vi "PV DATA TYPE.vi"(4 "String in":string, 5 "Data Typ String in":string) -> (1 "Substring":string, 2 "PV Protocol Data out":string)   [LabVIEW 2015, in "Pfeiffer Vacuum.lvlib"]
uses:
  Pfeiffer Vacuum.lvlib
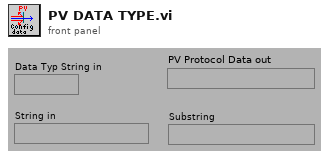
[diagram p1: front panel]
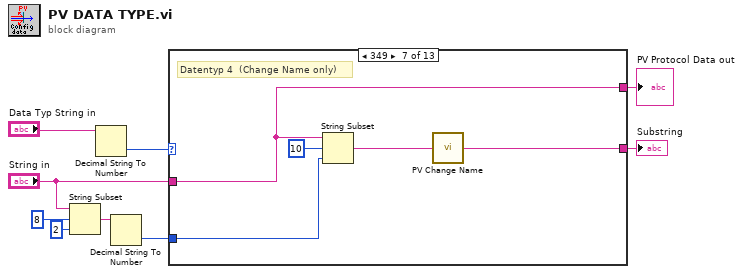
[diagram p0: block diagram]
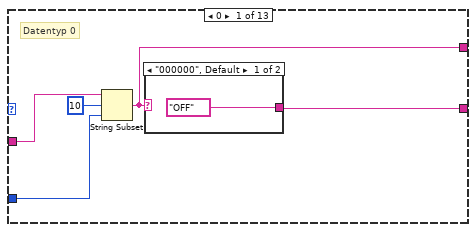
[diagram p2: hidden frame]
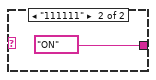
[diagram p3: hidden frame]
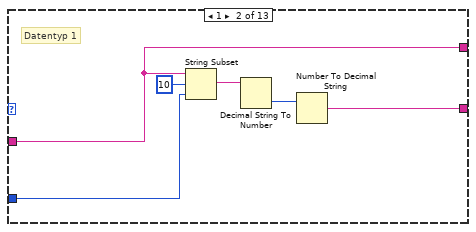
[diagram p4: hidden frame]
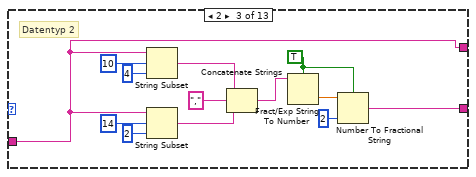
[diagram p5: hidden frame]
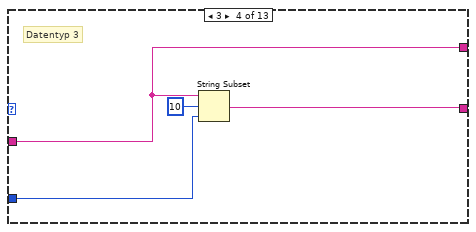
[diagram p6: hidden frame]
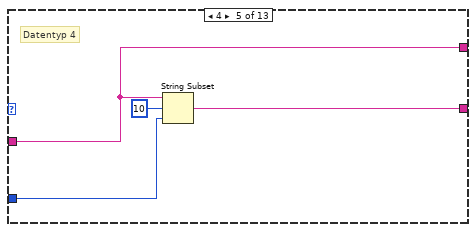
[diagram p7: hidden frame]
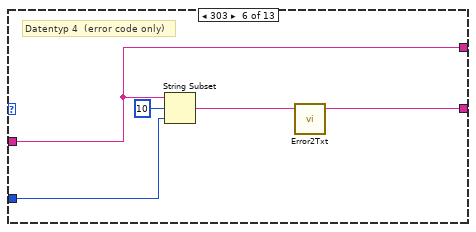
[diagram p8: hidden frame]
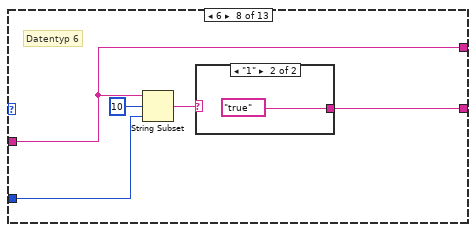
[diagram p9: hidden frame]
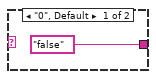
[diagram p10: hidden frame]
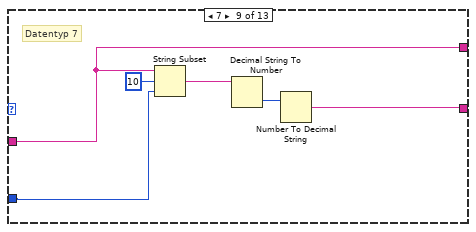
[diagram p11: hidden frame]
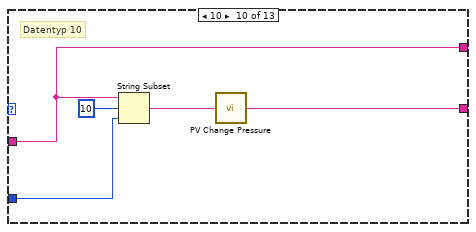
[diagram p12: hidden frame]
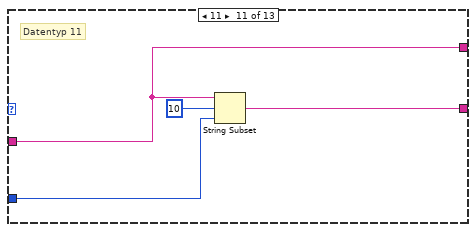
[diagram p13: hidden frame]
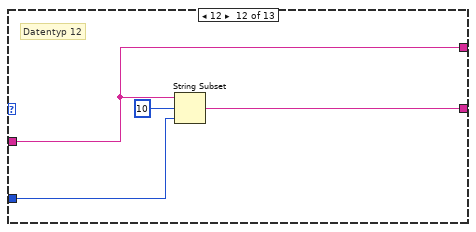
[diagram p14: hidden frame]
diagram:
  n1 = String Subset(string="String in", offset (0)=8 ("Offset (0)"), length (rest)=2 ("Länge (Rest)")) -> (substring=w4:string)
  n2 = Decimal String To Number(string="Data Typ String in") -> (number=w8:i32)  [unwired: 2 in, 1 out]
  n3 = Decimal String To Number(string=w4) -> (number=w2:i32)  [unwired: 2 in, 1 out]
  n4 = case shown="349" w8 {
    tunnel: "String in" -> [w12 w17 w23 w36 w40 w44 w49 w54 w61 w67 w72 w76 w80]
    tunnel: [w14 w21 w33 w38 w42 w46 w51 w56 w63 w69 w74 w77 w80] -> w9
    tunnel: w2 -> [w11 w18 _ w37 w41 w45 w50 w55 w62 w68 w73 w79 _]
    tunnel: [w10 w17 w23 w36 w40 w44 w49 w54 w61 w67 w72 w76 w80] -> w1
    frame 0 {
      # "Datentyp 0"
      n5 = String Subset(string=w12, offset (0)=10 ("Offset (0)"), length (rest)=w11) -> (substring=w10:string)
      n6 = case shown="\"000000\", Default" w10 {
        tunnel: ["OFF" "ON"] -> w14
        frame "000000", Default {
        }
        frame "111111" {
        }
      }
    }
    frame 1 {
      # "Datentyp 1"
      n7 = String Subset(string=w17, offset (0)=10 ("Offset (0)"), length (rest)=w18) -> (substring=w20:string)
      n8 = Decimal String To Number(string=w20) -> (number=w19:i32)  [unwired: 2 in, 1 out]
      n9 = Number To Decimal String(number=w19) -> (decimal integer string=w21:string)  [unwired: 1 in]
    }
    frame 2 {
      w24 = TRUE ("verwende System-Dezimalpunkt (T)")
      # "Datentyp 2"
      n10 = String Subset(string=w23, offset (0)=10 ("Offset (0)"), length (rest)=4 ("Länge")) -> (substring=w29:string)
      n11 = String Subset(string=w23, offset (0)=14 ("Offset (0)"), length (rest)=2 ("Länge")) -> (substring=w28:string)
      n12 = Concatenate Strings(w29, ",", w28) -> (w26:string)
      n13 = Fract/Exp String To Number(use system decimal point (T)=w24, string=w26) -> (number=w25:dbl)  [unwired: 2 in, 1 out]
      n14 = Number To Fractional String(use system decimal point (T)=w24, number=w25, precision (6)=i16 2 ("Genauigkeit (6)")) -> (F-format string=w33:string)  [unwired: 1 in]
    }
    frame 3 {
      # "Datentyp 3"
      n15 = String Subset(string=w36, offset (0)=10 ("Offset (0)"), length (rest)=w37) -> (substring=w38:string)
    }
    frame 4 {
      # "Datentyp 4"
      n16 = String Subset(string=w40, offset (0)=10 ("Offset (0)"), length (rest)=w41) -> (substring=w42:string)
    }
    frame 303 {
      # "Datentyp 4  (error code only)"
      n17 = String Subset(string=w44, offset (0)=10 ("Offset (0)"), length (rest)=w45) -> (substring=w47:string)
      n18 = call "Error2Txt.vi"("Error in"=w47) -> ("Description out"=w46:string)  [unwired: 4 in]
    }
    frame 349 {
      # "Datentyp 4  (Change Name only)"
      n19 = String Subset(string=w49, offset (0)=10 ("Offset (0)"), length (rest)=w50) -> (substring=w52:string)
      n20 = call "PV Change Name.vi"("Input"=w52) -> ("Output"=w51:string)
    }
    frame 6 {
      # "Datentyp 6"
      n21 = String Subset(string=w54, offset (0)=10 ("Offset (0)"), length (rest)=w55) -> (substring=w57:string)
      n22 = case shown="\"1\"" w57 {
        tunnel: ["false" "true"] -> w56
        frame "0", Default {
        }
        frame "1" {
        }
      }
    }
    frame 7 {
      # "Datentyp 7"
      n23 = String Subset(string=w61, offset (0)=10 ("Offset (0)"), length (rest)=w62) -> (substring=w64:string)
      n24 = Decimal String To Number(string=w64) -> (number=w65:i32)  [unwired: 2 in, 1 out]
      n25 = Number To Decimal String(number=w65) -> (decimal integer string=w63:string)  [unwired: 1 in]
    }
    frame 10 {
      # "Datentyp 10"
      n26 = String Subset(string=w67, offset (0)=10 ("Offset (0)"), length (rest)=w68) -> (substring=w70:string)
      n27 = call "PV Change Pressure.vi"("Pressure String"=w70) -> ("Change Pressure String"=w69:string)
    }
    frame 11 {
      # "Datentyp 11"
      n28 = String Subset(string=w72, offset (0)=10 ("Offset (0)"), length (rest)=w73) -> (substring=w74:string)
    }
    frame 12 {
      # "Datentyp 12"
      n29 = String Subset(string=w76, offset (0)=10 ("Offset (0)"), length (rest)=w79) -> (substring=w77:string)
    }
    frame Default {
    }
  }
  "Substring" <- w9
  "PV Protocol Data out" <- w1
